vi "forceaboutplane.vi"() -> ()   [LabVIEW 2017]
panel:
  in  "angles":dbl[](array[numeric])
  in  "K constant_pel":dbl
  in  "pel_cn_atStanding":dbl[](array[numeric])
  in  "viconData_2":dbl[](array[numeric])
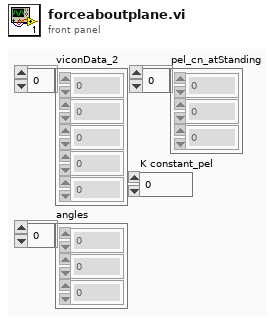
[diagram p1: front panel]
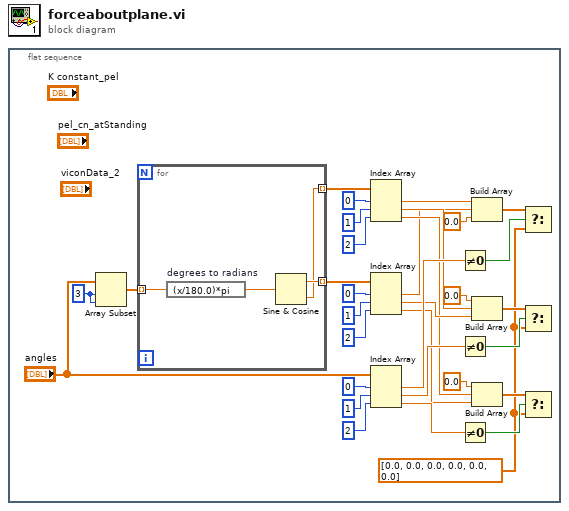
[diagram p0: block diagram]
diagram:
  n1 = flat-sequence {
    frame #0 {
      w25 = 3 ("index")
      w1 = dbl[] [0.0, 0.0, 0.0, 0.0, 0.0, 0.0]
      n2 = Array Subset(array="angles", index=w25, length=w25) -> (w24:dbl[])
      n3 = for {
        tunnel: w24 -> [w36] mode=indexing
        tunnel: [w35] -> w22 mode=indexing
        tunnel: [w34] -> w13 mode=indexing
        n4 = expression code="(x/180.0)*pi" "degrees to radians"(w36) -> (w37:dbl)
        n5 = Sine & Cosine(0:w37) -> (1:w35:dbl, 2:w34:dbl)
      }
      n6 = Index Array(array=w13, index #1=0 ("index"), index #2=1 ("index"), index #3=2 ("index")) -> (element #1=w5:dbl, element #2=w12:dbl, element #3=w10:dbl)
      n7 = Index Array(array=w22, index #1=0 ("index"), index #2=1 ("index"), index #3=2 ("index")) -> (element #1=w4:dbl, element #2=w18:dbl, element #3=w9:dbl)
      n8 = Index Array(array="angles", index #1=0 ("index"), index #2=1 ("index"), index #3=2 ("index")) -> (element #1=w32:dbl, element #2=w29:dbl, element #3=w28:dbl)
      n9 = Not Equal To 0?(x=w32) -> (x != 0?=w3:bool)
      n10 = Not Equal To 0?(x=w29) -> (x != 0?=w27:bool)
      n11 = Not Equal To 0?(x=w28) -> (x != 0?=w8:bool)
      n12 = Build Array(w5, w4, 0.0 ("element")) -> (w2:dbl[])
      n13 = Build Array(0.0 ("element"), w12, w18) -> (w11:dbl[])
      n14 = Build Array(0.0 ("element"), w10, w9) -> (w7:dbl[])
      n15 = Select(t=w2, s=w3, f=w1) -> ()  [unwired: 1 out]
      n16 = Select(t=w11, s=w27, f=w1) -> ()  [unwired: 1 out]
      n17 = Select(t=w7, s=w8, f=w1) -> ()  [unwired: 1 out]
    }
  }
